vi "Global_CMD_ACT_Data In.vi"() -> ()   [LabVIEW 2020, in "Arm_ACT.lvlib"]
uses:
  Arm_ACT.lvlib
  Cluster_CMD_ACT_Data.ctl
panel:
  in  "CMD_ACT_Template_Data":T1
  # "The Names of the Data items in the Global Variable MUST describe who the Single Writer is\nFor Command Globals the Commander(CMD) represents Teleop or Autonomous or other command loop.\nThe naming convention for a Command Actuator Global is:   \n\nCMD_ACT_SubSystem_Data Name\n\nExample:\nCMD_ACT_Drive_Data\nCMD_ACT_Hopper_Eject Ball"
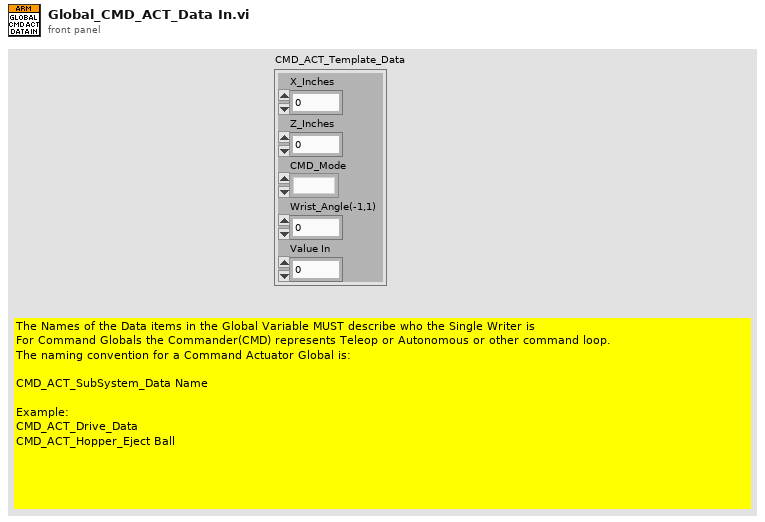
[diagram p1: front panel]
types:
  T1 = typedef "Arm_ACT.lvlib/Cluster_CMD_ACT_Data.ctl" = cluster{"X_Inches":dbl, "Z_Inches":dbl, "CMD_Mode":enum16{""}, "Wrist_Angle(-1,1)":dbl, "Value In":dbl}
diagram:
